vi "Lock In Amplifier Status.vi"(8 "error in (no error)":errorcluster, 11 "VISA resource name":refnum<visa-resource-name>) -> (0 "error out":errorcluster, 2 "Lock In Amplifier Data Message":string, 3 "VISA resource name out":refnum<visa-resource-name>, 5 "Time overload":bool, 6 "Input":bool, 7 "output overload":bool)   [LabVIEW 2017]
doc: "Queries the Lock-In Amplifier Status register for the Questionable Data Register group. Essentially, it is used to observe possible invalid results."
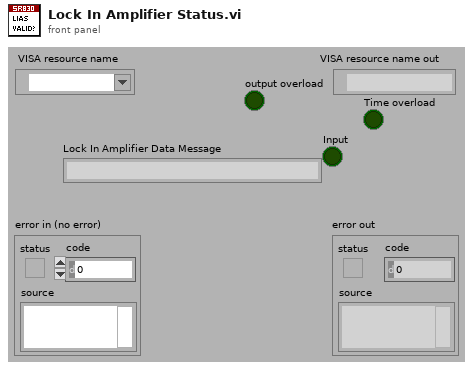
[diagram p1: front panel]
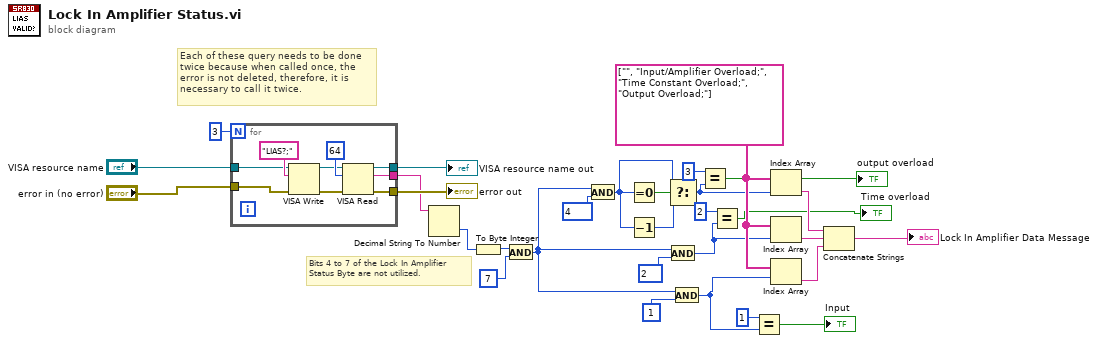
[diagram p0: block diagram]
diagram:
  w28 = string[] ["", "Input/Amplifier Overload;", "Time Constant Overload;", "Output Overload;"]
  # "Each of these query needs to be done twice because when called once, the error is not deleted, therefore, it is necessary to call it twice."
  # "Bits 4 to 7 of the Lock In Amplifier Status Byte are not utilized."
  n1 = for {
    N: 3 -> [_]
    tunnel: [w35] -> w15
    tunnel: [w34] -> w14
    tunnel: [w33] -> w13
    tunnel: "VISA resource name" -> [w32]
    tunnel: "error in (no error)" -> [w31]
    n2 = VISA Write(VISA resource name=w32, write buffer="LIAS?;", error in (no error)=w31) -> (VISA resource name out=w37:refnum<visa-resource-name>, error out=w36:errorcluster)  [unwired: 1 out]
    n3 = VISA Read(VISA resource name=w37, byte count=u32 64, error in (no error)=w36) -> (VISA resource name out=w35:refnum<visa-resource-name>, read buffer=w33:string, error out=w34:errorcluster)  [unwired: 1 out]
  }
  "error out" <- w14
  "VISA resource name out" <- w15
  n4 = Decimal String To Number(string=w13) -> (number=w30:i32)  [unwired: 2 in, 1 out]
  n5 = To Byte Integer(number=w30) -> (8bit integer=w27:i8)
  n6 = And(x=w27, y=i8 7 ("value")) -> (x .and. y?=w16:i8)
  n7 = And(x=w16, y=i8 4) -> (x .and. y?=w20:i8)
  n8 = Equal To 0?(x=w20) -> (x = 0?=w22:bool)
  n9 = Decrement(x=w20) -> (x-1=w21:i8)
  n10 = Select(t=w20, s=w22, f=w21) -> (s? t:f=w12:i8)
  n11 = And(x=w16, y=i8 2) -> (x .and. y?=w8:i8)
  n12 = And(x=w16, y=i8 1) -> (x .and. y?=w5:i8)
  n13 = Equal?(x=i8 3, y=w12) -> (x = y?=→"output overload":bool)
  n14 = Equal?(x=i8 2, y=w8) -> (x = y?=→"Time overload":bool)
  n15 = Equal?(x=i8 1, y=w5) -> (x = y?=→"Input":bool)
  n16 = Index Array(array=w28, index=w12) -> (element=w23:string)
  n17 = Index Array(array=w28, index=w8) -> (element=w18:string)
  n18 = Index Array(array=w28, index=w5) -> (element=w17:string)
  n19 = Concatenate Strings(w23, w18, w17) -> (→"Lock In Amplifier Data Message":string)
